vi "Build-image-label.vi"(6 "Image #":i32, 8 "error in":errorcluster, 9 "Image label":string, 10 "Base file name":string) -> (0 "error IO":errorcluster, 2 "Filename":string)   [LabVIEW 2013, in "CameraVision.lvlib" / "CV-Storage.lvclass"]
uses:
  CV-Storage.lvclass
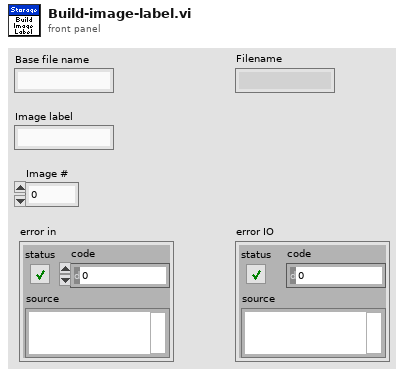
[diagram p1: front panel]
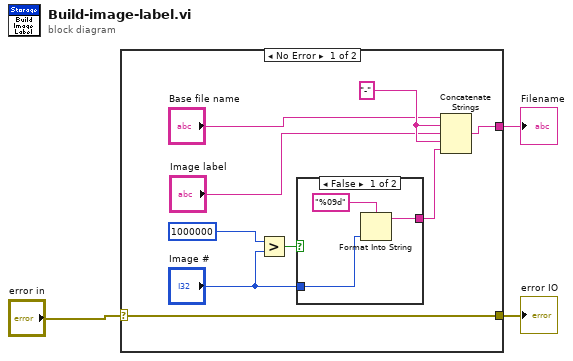
[diagram p0: block diagram]
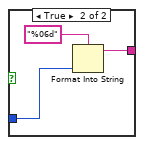
[diagram p2: hidden frame]
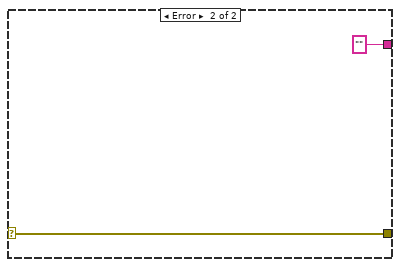
[diagram p3: hidden frame]
diagram:
  n1 = case shown="No Error" "error in" {
    selector: "error in" -> [w7 w19]
    tunnel: [w8 ""] -> w3
    tunnel: [w7 w19] -> w1
    frame No Error {
      w12 = "-" ("string")
      n2 = Greater?(x=1000000, y="Image #") -> (0:w6:bool)
      n3 = case shown="False" w6 {
        tunnel: "Image #" -> [w15 w18]
        tunnel: [w14 w16] -> w9
        frame False {
          n4 = Format Into String(format string="%09d", w15) -> (resulting string=w14:string)  [unwired: 2 in, 1 out]
        }
        frame True {
          n5 = Format Into String(format string="%06d", w18) -> (resulting string=w16:string)  [unwired: 2 in, 1 out]
        }
      }
      n6 = Concatenate Strings("Base file name", w12, "Image label", w12, w9) -> (w8:string)
    }
    frame Error {
    }
  }
  "Filename" <- w3
  "error IO" <- w1
